vi "GetExternalInterfaces.vi"(8 "ErrorIn":errorcluster, 11 "ObjectIn":refnum<class "ITAFObject.lvclass">) -> (0 "ErrorOut":errorcluster, 2 "ExternalInterfaces":T1[](array[typedef]), 3 "ObjectOut":refnum<class "ITAFObject.lvclass">)   [LabVIEW 2021, in "ITAFObject.lvclass"]
uses:
  ITAFObject.lvclass
  Library_TAF_Support/ClusterArrayConversion/BundledArray.ctl
  Library_TAF_Support/ClusterArrayConversion/ClusterArrayConversion.lvlib
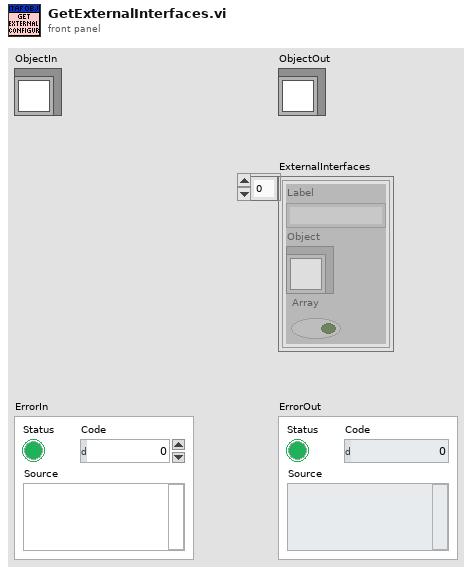
[diagram p1: front panel]
types:
  T1 = typedef "ClusterArrayConversion.lvlib/BundledArray.ctl" = cluster{"Label":string, "Object":refnum<class>, "Array":bool}
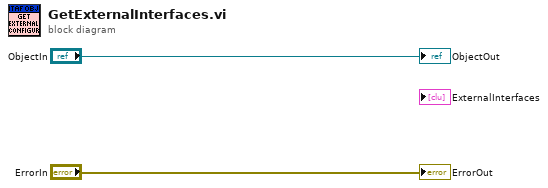
[diagram p0: block diagram]
diagram:
  "ErrorOut" <- "ErrorIn"
  "ObjectOut" <- "ObjectIn"
